vi "FGV_Obtain Multi bin file paths and refs.vi"(8 "error in (no error)":errorcluster, 10 "Function":T1, 11 "Timelapse folder path":path) -> (0 "Error out":errorcluster, 2 "Cam Binary Videos":path[](array[path]))   [LabVIEW 2017]
uses:
  Functional Imaging Viewer/Typedefs/Get-Set-Clear Control.ctl
  <userlib>/_OpenG.lib/array/array.llb/Conditional Auto-Indexing Tunnel (Path)__ogtk.vi
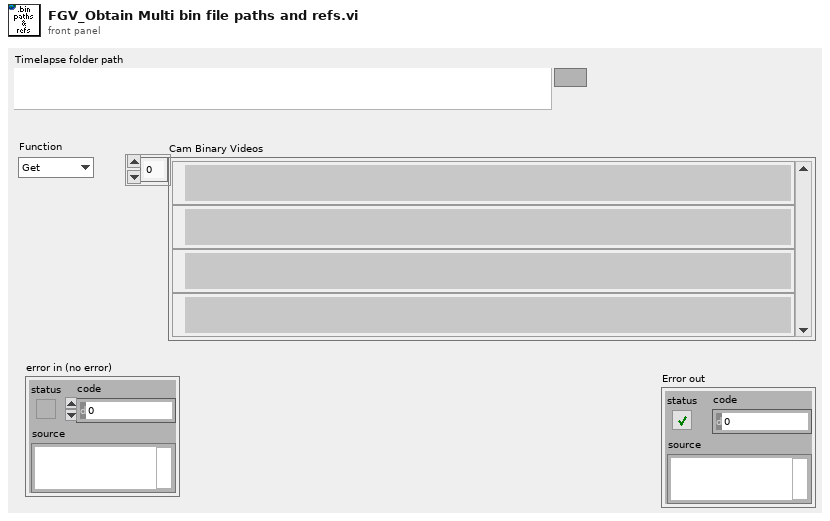
[diagram p1: front panel]
types:
  T1 = typedef "Get-Set-Clear Control.ctl" = enum16{"Get", "Set", "Clear"}
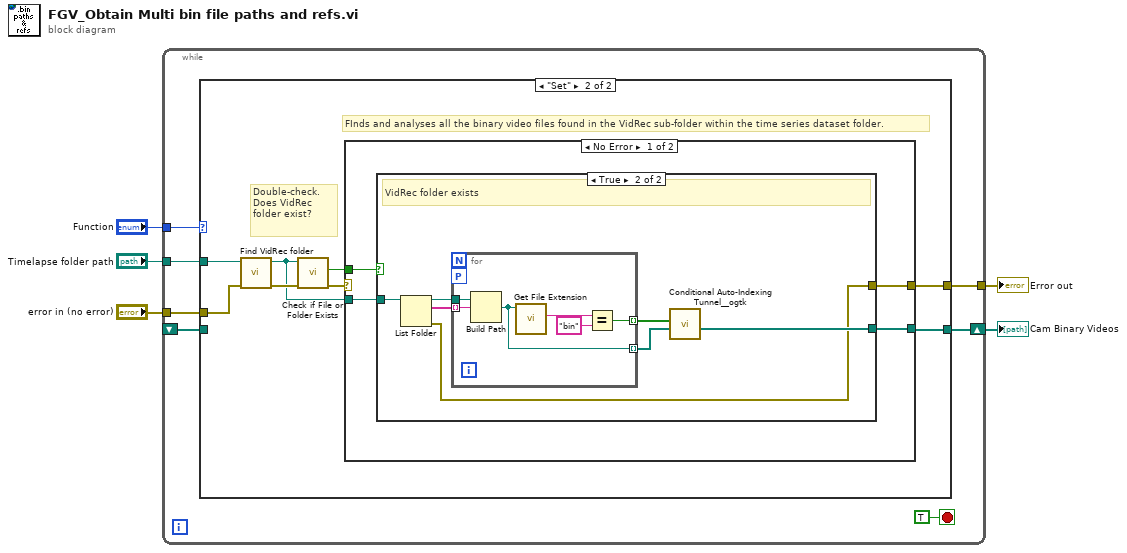
[diagram p0: block diagram]
diagram:
  n1 = while {
    tunnel: "Timelapse folder path" -> [w12]
    tunnel: [w11] -> w1
    tunnel: "error in (no error)" -> [w9]
    tunnel: "Function" -> [w7]
    shift-right: [w10] -> w2
    shift-left: _ -> [w6]
    stop <- TRUE stop-if-true
    n2 = case shown="\"Set\"" w7 {
      tunnel: w12 -> [_ w18]
      tunnel: [w14 w20] -> w11
      tunnel: [w13 w19] -> w10
      tunnel: w9 -> [w14 w17]
      tunnel: w6 -> [w13 _]
      frame "Get", Default {
      }
      frame "Set" {
        # "FInds and analyses all the binary video files found in the VidRec sub-folder within the time series dataset folder."
        # "Double-check.\nDoes VidRec folder exist?"
        n3 = call "Find VidRec folder.vi"("error in (no error)"=w17, "Timelapse folder path"=w18) -> ("error out"=w16:errorcluster, "appended path"=w15:path)  [unwired: 8 in]
        n4 = call <vilib>:"Check if File or Folder Exists.vi"("error in (no error)"=w16, "path"=w15) -> ("error out"=w21:errorcluster, "file or folder exists?"=w22:bool)  [unwired: 7 in, 1 out]
        n5 = case shown="No Error" w21 {
          selector: w21 -> [_ w40]
          tunnel: w22 -> [w26 _]
          tunnel: w15 -> [w25 _]
          tunnel: [w23 w40] -> w20
          tunnel: [w24 _] -> w19
          frame No Error {
            n6 = case shown="True" w26 {
              tunnel: w25 -> [_ w33]
              tunnel: [_ w28] -> w24
              tunnel: [_ w27] -> w23
              frame False {
                # "VidRec folder does not exist"
              }
              frame True {
                # "VidRec folder exists"
                n7 = List Folder(path=w33) -> (path out=w31:path, filenames=w32:string[], error out=w27:errorcluster)  [unwired: 3 in, 1 out]
                n8 = for {
                  tunnel: w32 -> [w38] mode=indexing
                  tunnel: w31 -> [w39]
                  tunnel: [w35] -> w30 mode=indexing
                  tunnel: [w34] -> w29 mode=indexing
                  workers-P: _ -> [_]
                  n9 = Build Path(base path=w39, name or relative path=w38) -> (appended path=w34:path)
                  n10 = call <vilib>:"Get File Extension.vi"("file"=w34) -> ("lowercase file extension"=w37:string)  [unwired: 6 in, 4 out]
                  n11 = Equal?(x=w37, y="bin") -> (x = y?=w35:bool)
                }
                n12 = call-poly <userlib>:"Conditional Auto-Indexing Tunnel__ogtk.vi"("Array in"=w29, "Elements to keep"=w30) -> ("Filtered Array out"=w28:path[])  [unwired: 5 in]
              }
            }
          }
          frame Error {
          }
        }
      }
    }
  }
  "Cam Binary Videos" <- w2
  "Error out" <- w1
